vi "Start Iteration.vi"(11 "Loop Data in":T1) -> (3 "Loop Data":T1)   [LabVIEW 2020, in "VolatusDaq.lvlib" / "DaqControl.lvclass"]
uses:
  DaqControl.lvclass
  Loop Data.ctl
  Volatus/Event API/EventAPI.lvclass
  Volatus/DataHandlerAPI/DataHandlerAPI.lvclass
  Sequence Action.ctl
  Seq Action Type.ctl
  Value Update.ctl
  Seq Cmd.ctl
  Seq Cmd Type.ctl
  Signal Type.ctl
  DaqControl.lvclass/DaqControl.ctl
  VolatusDaq.lvlib
  Sequence.ctl
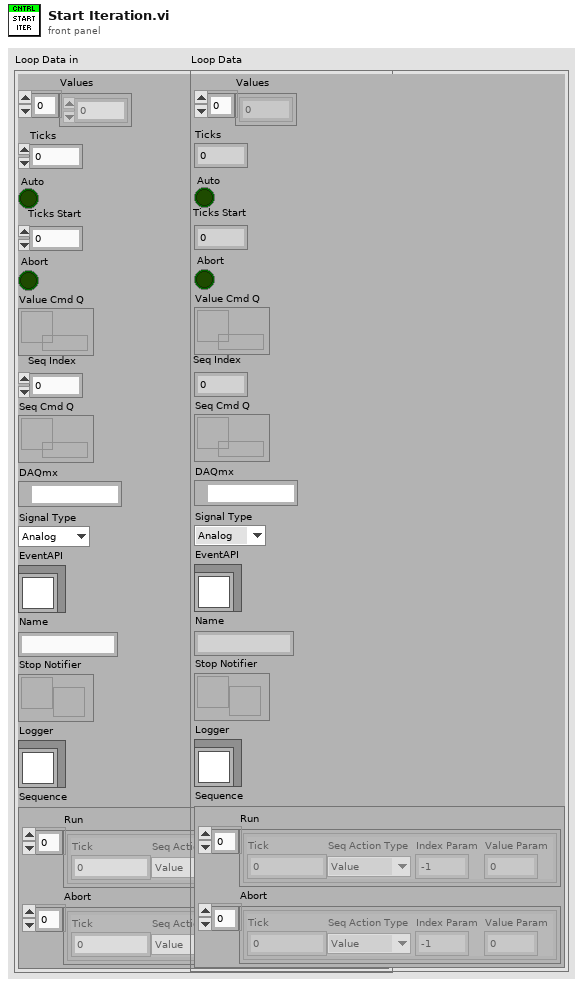
[diagram p1: front panel]
types:
  T1 = typedef "VolatusDaq.lvlib/DaqControl.lvclass/Loop Data.ctl" = cluster{"Values":dbl[], "Ticks":u32, "Auto":bool, "Ticks Start":u32, "Abort":bool, "Value Cmd Q":refnum<queue>, "Seq Index":i32, "Seq Cmd Q":refnum<queue>, "DAQmx":refnum<k21>, "Signal Type":T2, "EventAPI":refnum<class "EventAPI.lvclass">, "Name":string, "Stop Notifier":refnum<notifier>, "Logger":refnum<class "DataHandlerAPI.lvclass">, "Sequence":T3}
  T2 = typedef "VolatusDaq.lvlib/Signal Type.ctl" = enum16{"Analog", "Digital"}
  T3 = typedef "VolatusDaq.lvlib/Sequence.ctl" = cluster{"Run":T4[], "Abort":T4[]}
  T4 = typedef "VolatusDaq.lvlib/Sequence Action.ctl" = cluster{"Tick":u32, "Seq Action Type":T5, "Index Param":i32, "Value Param":dbl}
  T5 = typedef "VolatusDaq.lvlib/Seq Action Type.ctl" = enum16{"Value", "Stop"}
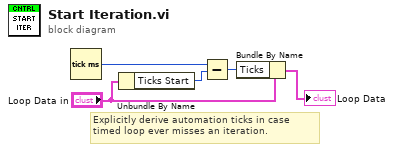
[diagram p0: block diagram]
diagram:
  # "Explicitly derive automation ticks in case timed loop ever misses an iteration."
  n1 = Tick Count (ms)() -> (millisecond timer value=w4:u32)
  n2 = Unbundle By Name("Loop Data in") -> ("Ticks Start"=w5:u32)
  n3 = Subtract(x=w4, y=w5) -> (x-y=w2:u32)
  n4 = Bundle By Name(cluster="Loop Data in", "Ticks"=w2) -> (→"Loop Data":T1)
